vi "sCMOS_ROI_extract.vi"(2 "Image IN":T1, 3 "ROI":T2, 4 "error in":errorcluster, 5 "Image ROI":T1) -> (0 "error out":errorcluster, 1 "Image Out":T1)   [LabVIEW 2015]
uses:
  <vilib>/vision/Image Controls.llb/IMAQ Image.ctl
  <vilib>/vision/NI_Vision_Development_Module.lvlib
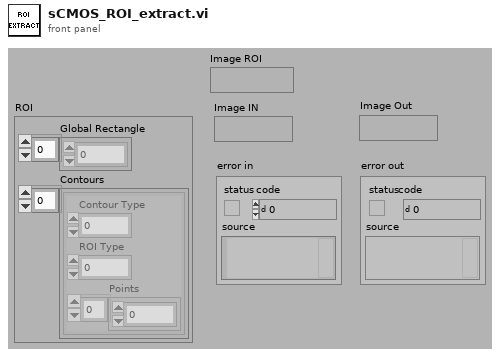
[diagram p1: front panel]
types:
  T1 = typedef "IMAQ Image.ctl" = refnum<image>
  T2 = cluster{"Global Rectangle":i32[], "Contours":cluster{"Contour Type":u32, "ROI Type":u32, "Points":i32[]}[]}
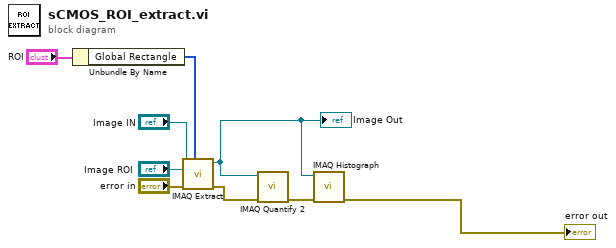
[diagram p0: block diagram]
diagram:
  n1 = Unbundle By Name("ROI") -> ("Global Rectangle"=w3:i32[])
  n2 = call "IMAQ Extract"("Optional Rectangle"=w3, "error in (no error)"="error in", "Image Dst"="Image ROI", "Image Src"="Image IN") -> ("error out"=w5:errorcluster, "Image Dst Out"=w6:T1)  [unwired: 6 in]
  "Image Out" <- w6
  n3 = call "IMAQ Quantify 2"("error in (no error)"=w5, "Image"=w6) -> ("error out"=w4:errorcluster)  [unwired: 7 in, 2 out]
  n4 = call "IMAQ Histograph"("error in (no error)"=w4, "Image"=w6) -> ("error out"=→"error out":errorcluster)  [unwired: 6 in, 3 out]
